vi "Sync_Afterwards.vi"(2 "Analogue Data":dbl[][](array[numeric]) format="%.3f", 4 "LDA Data":dbl[][](array[numeric]) format="%.3f") -> (0 "Eng Values":dbl[][](array[numeric]) format="%.2f")   [LabVIEW 2011]
uses:
  Globals/LDA_meas_global_1.vi
  Globals/Meas_global.vi
  Globals/Dynamic_call_global.ph.vi
panel:
  out "Array":string[](array[string])
  out "Delay (ms)":dbl=13.0 format="%.2f"
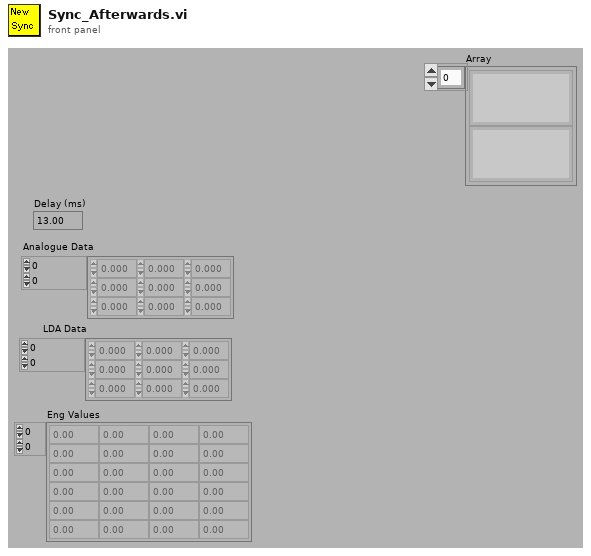
[diagram p1: front panel]
types:
  T1 = typedef "Analysis_info_cluster.ctl" = cluster{"Colour":u32, "Inst type":T2, "Inst name":string, "Symbol":string, "Code name":string, "Extra Info":string, "Inst Array":T3, "Index":i32, "Voltage Index":i32, "Extra Titles":string[], "Extra Values":string[], "Eng Values":dbl[], "Time (ms)":dbl[], "TT / Voltage":dbl[], "U":dbl, "u^2":dbl, "u^3":dbl, "u^4":dbl, "Skew_u":dbl, "Kurt_u":dbl, "Mean % Err":dbl, "% u'/U":dbl}
  T2 = typedef "Inst_type.ctl" = enum16{"Propeller anemometer", "Raw voltage", "Pressure Transducer", "Pitot-static tube", "Preston tube", "Hot wire", "Cross wire 1", "Cross wire 2", "Generic Linear", "Generic Polynomial", "Generic BackPoly", "Fast FID", "Thermocouple", "Cold wire", "Pulsed Wire", "LDA Vel", "LDA Tran time", "LDA Arr time"}
  T3 = typedef "Instrument_Array.ctl" = enum16{"PWA", "LDA", "Analogue"}
  T4 = typedef "Analysis_type_cluster.ctl" = cluster{"Analysis type":T5, "Indicies":i32[], "Name":string, "Inst Array":T3, "Info index":i32}
  T5 = typedef "Analysis_type_Enum.ctl" = enum16{"Slow Response", "Fast Response", "Weighted Fast Response", "Fast FID", "Weighted Fast FID", "Cross Wire", "Weighted Cross Wire", "Weighted LDA"}
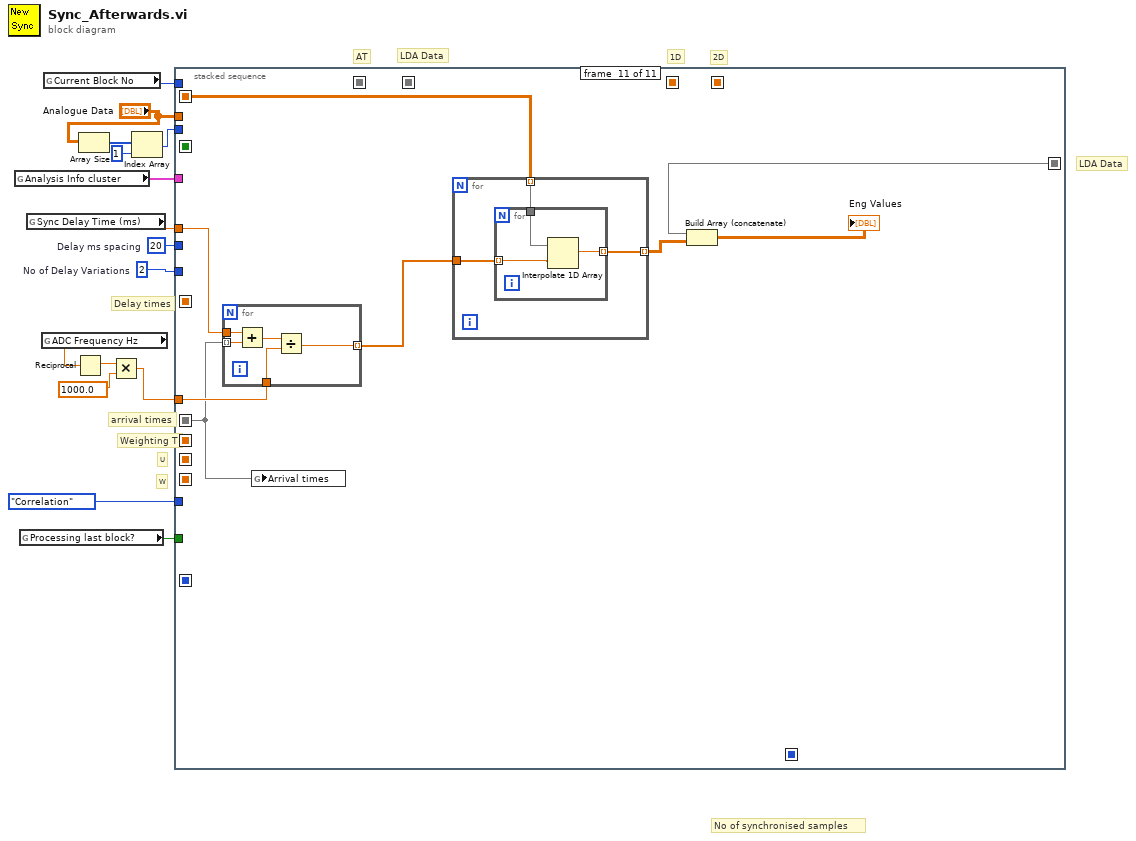
[diagram p0: block diagram]
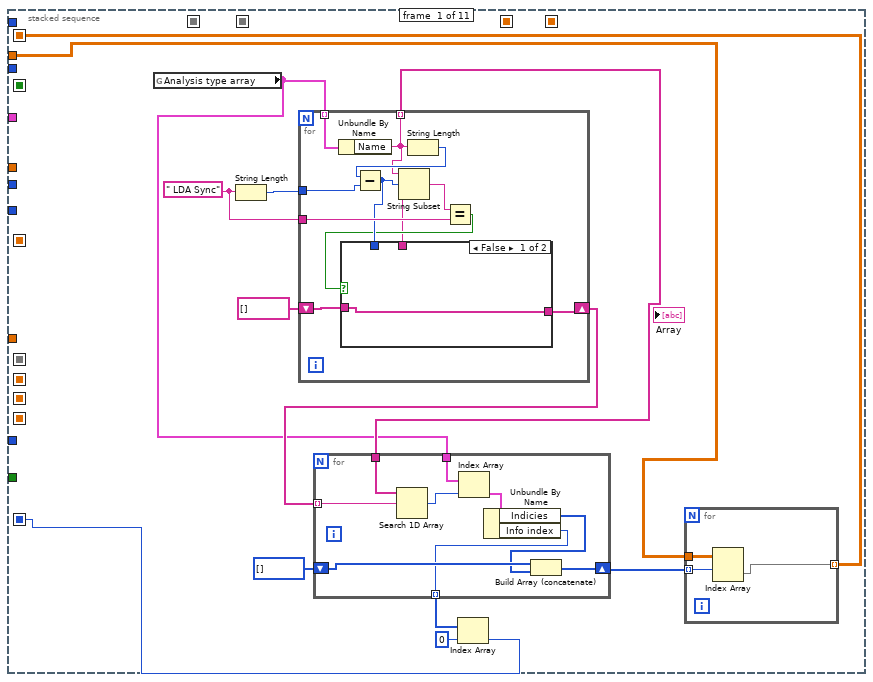
[diagram p2: hidden frame]
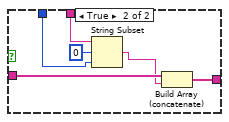
[diagram p3: hidden frame]
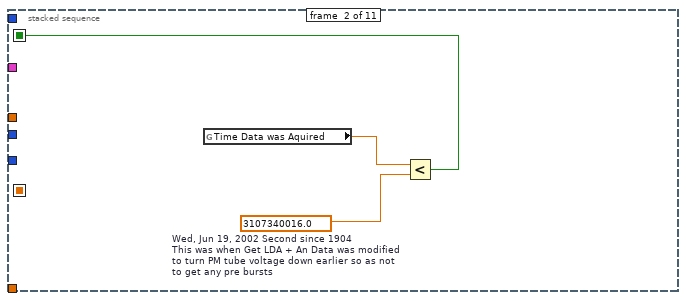
[diagram p4: hidden frame]
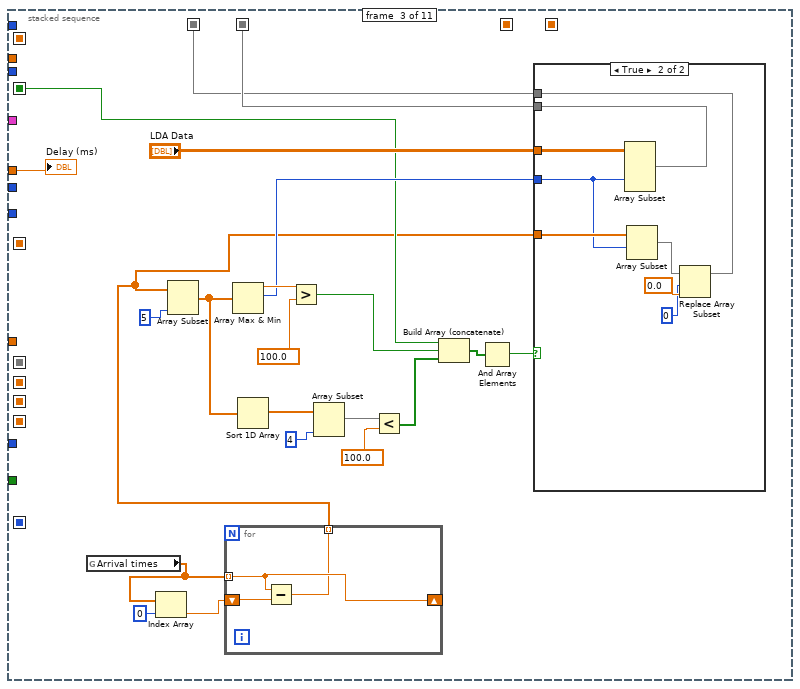
[diagram p5: hidden frame]
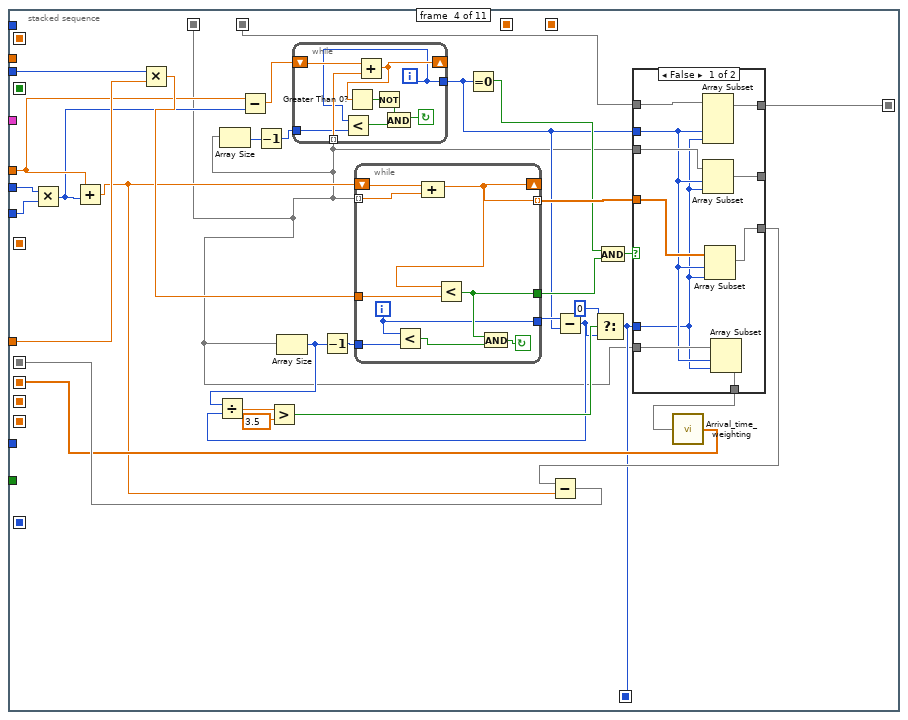
[diagram p7: hidden frame]
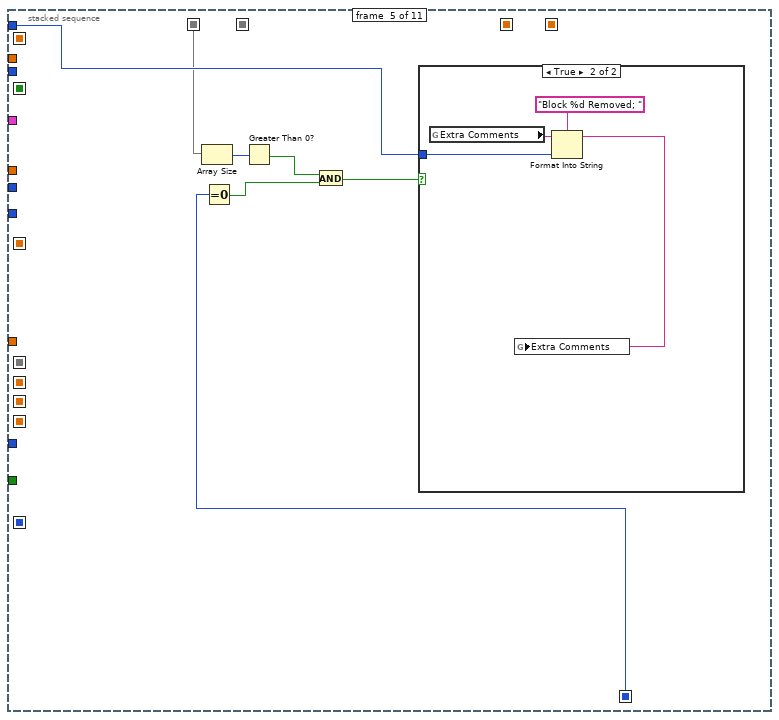
[diagram p9: hidden frame]
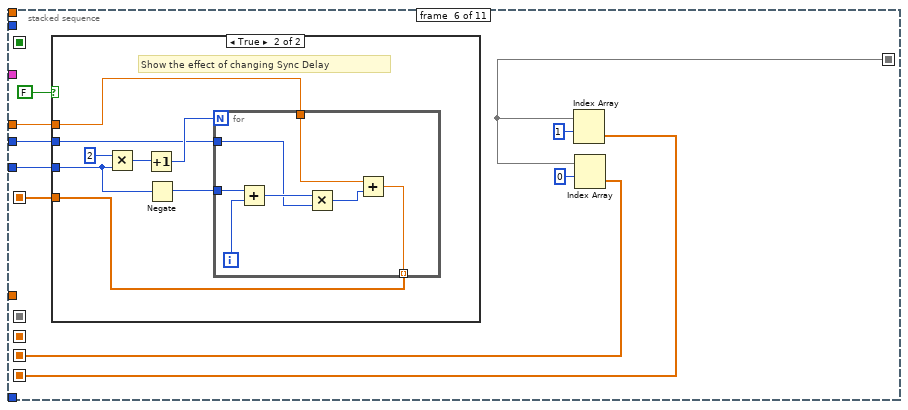
[diagram p11: hidden frame]
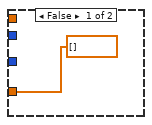
[diagram p12: hidden frame]
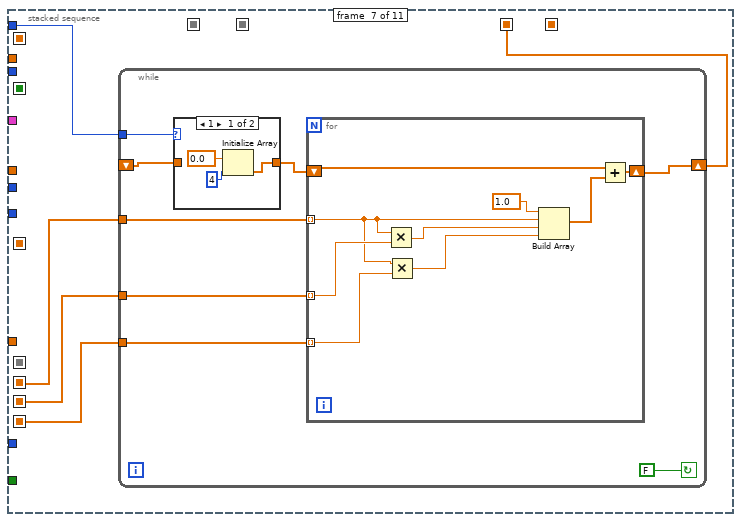
[diagram p13: hidden frame]
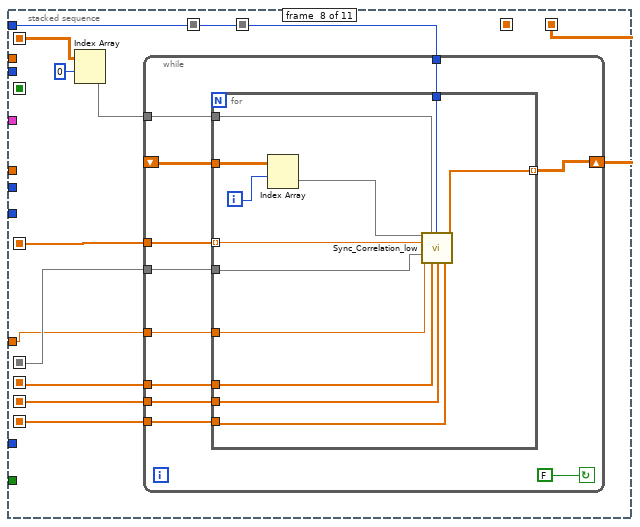
[diagram p15: hidden frame]
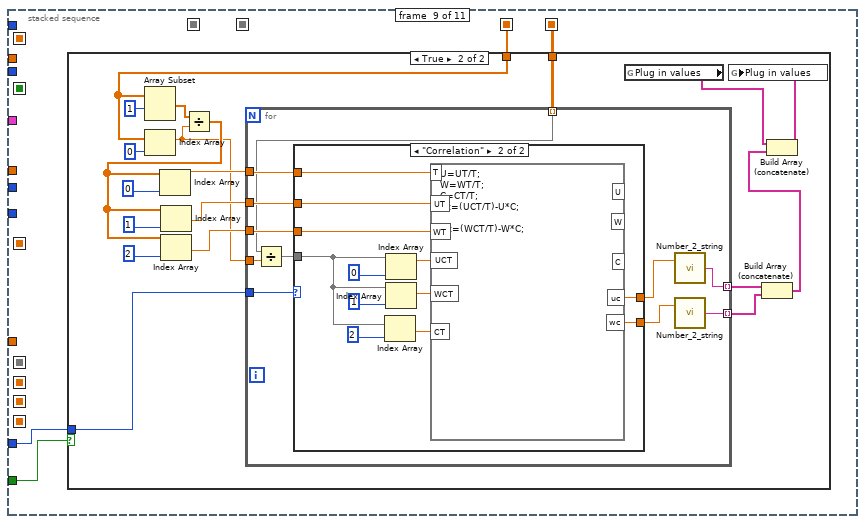
[diagram p16: hidden frame]
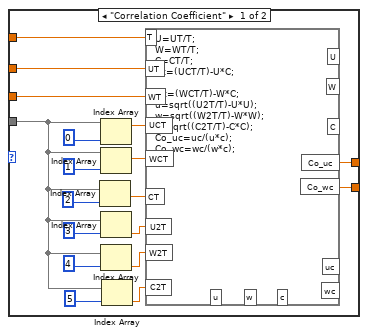
[diagram p18: hidden frame]
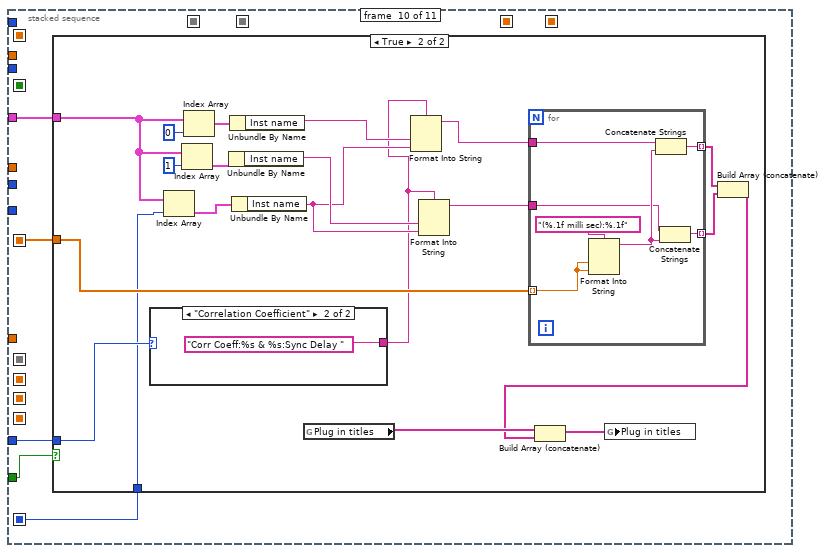
[diagram p19: hidden frame]
diagram:
  w3 = 20  # Delay ms spacing
  w15 = 2  # No of Delay Variations
  # "No of synchronised samples"
  # "AT"
  # "LDA Data"
  # "Delay times"
  # "1D"
  # "2D"
  # "W"
  # "U"
  # "Weighting T"
  # "arrival times"
  # "LDA Data"
  n1 = global read "Meas_global.vi" "Analysis Info cluster"() -> (w1:T1[])
  n2 = global read "Meas_global.vi" "Processing last block?"() -> (w13:bool)
  n3 = global read "LDA_meas_global_1.vi" "Sync Delay Time (ms)"() -> (w8:dbl)
  n4 = global read "LDA_meas_global_1.vi" "ADC Frequency Hz"() -> (w11:dbl)
  n5 = global read "Meas_global.vi" "Current Block No"() -> (w14:i32)
  n6 = Reciprocal(x=w11) -> (1/x=w12:dbl)
  n7 = Array Size(array="Analogue Data") -> (size(s)=w6:i32[])
  n8 = Multiply(x=w12, y=1000.0) -> (x*y=w9:dbl)
  n9 = Index Array(array=w6, index=1 ("Index")) -> (element=w4:i32)
  n10 = stacked-sequence {
    seq-local: [_ _ _ w125 _ _ _ _ _ _ _] -> [_ _ _ _ _ w176 _ _ _ _ w360]
    seq-local: [_ _ _ w122 _ _ _ _ _ _ _] -> [_ _ _ _ _ _ _ w228 _ _ w355]
    seq-local: [_ _ _ w120 _ _ _ _ _ _ _] -> [_ _ _ _ _ _ w201 w229 _ _ _]
    seq-local: [_ _ _ _ _ w175 _ _ _ _ _] -> [_ _ _ _ _ _ w200 w231 _ _ _]
    seq-local: [_ _ _ _ _ w174 _ _ _ _ _] -> [_ _ _ _ _ _ w199 w230 _ _ _]
    seq-local: [_ _ _ _ _ _ _ w226 _ _ _] -> [_ _ _ _ _ _ _ _ w258 _ _]
    seq-local: [_ _ _ _ _ _ w197 _ _ _ _] -> [_ _ _ _ _ _ _ _ w259 _ _]
    seq-local: [_ _ _ _ _ w179 _ _ _ _ _] -> [_ _ _ _ _ _ _ w225 _ w324 _]
    seq-local: [_ _ w69 _ _ _ _ _ _ _ _] -> [_ _ _ w112 _ _ _ _ _ _ _]
    seq-local: [_ _ w68 _ _ _ _ _ _ _ _] -> [_ _ _ w98 w165 _ _ _ _ _ _]
    seq-local: [_ w59 _ _ _ _ _ _ _ _ _] -> [_ _ w65 _ _ _ _ _ _ _ _]
    seq-local: [_ _ _ w102 _ _ _ _ _ _ _] -> [_ _ _ _ w164 _ _ _ _ _ _]
    seq-local: [w17 _ _ _ _ _ _ _ _ _ _] -> [_ _ _ _ _ _ _ _ _ w321 _]
    seq-local: [w16 _ _ _ _ _ _ _ _ _ _] -> [_ _ _ _ _ _ _ w223 _ _ w357]
    tunnel: "Analogue Data" -> [w20 _ _ _ _ _ _ _ _ _ _]
    tunnel: w8 -> [_ _ w66 w114 _ w173 _ _ _ _ w356]
    tunnel: w15 -> [_ _ _ w100 _ w180 _ _ _ _ _]
    tunnel: w14 -> [_ _ _ _ w166 _ w198 w227 _ _ _]
    tunnel: w13 -> [_ _ _ _ _ _ _ _ w260 w325 _]
    tunnel: w9 -> [_ _ _ w119 _ _ _ w224 _ _ w362]
    tunnel: w4 -> [_ _ _ w104 _ _ _ _ _ _ _]
    tunnel: w3 -> [_ _ _ w101 _ w172 _ _ _ _ _]
    tunnel: enum16{"Correlation", "Correlation Coefficient"}."Correlation" -> [_ _ _ _ _ _ _ _ w257 w323 _]
    tunnel: w1 -> [_ _ _ _ _ _ _ _ _ w322 _]
    frame #0 {
      w27 = " LDA Sync" ("Substring")
      n11 = global read "Meas_global.vi" "Analysis type array"() -> (w23:T4[])
      n12 = String Length(string=w27) -> (length=w26:i32)
      n13 = for {
        tunnel: w23 -> [w50] mode=indexing
        tunnel: w26 -> [w48]
        tunnel: w27 -> [w46]
        shift-right: [w42] -> w24
        shift-left: string[] [] -> [w43]
        tunnel: [w41] -> w25 mode=indexing
        n14 = Unbundle By Name(w50) -> ("Name"=w41:string)
        n15 = String Length(string=w41) -> (length=w49:i32)
        n16 = Subtract(x=w49, y=w48) -> (x-y=w45:i32)
        n17 = String Subset(string=w41, offset (0)=w45) -> (substring=w47:string)  [unwired: 1 out]
        n18 = Equal?(x=w47, y=w46) -> (x = y?=w44:bool)
        n19 = case shown="False" w44 {
          tunnel: w41 -> [_ w57]
          tunnel: w45 -> [_ w55]
          tunnel: w43 -> [w51 w54]
          tunnel: [w51 w52] -> w42
          frame False {
          }
          frame True {
            n20 = String Subset(string=w57, offset (0)=0, length (rest)=w55) -> (substring=w53:string)
            n21 = Build Array (concatenate)(w54, w53) -> (w52:string[])
          }
        }
      }
      n22 = for {
        tunnel: w25 -> [w40]
        tunnel: w24 -> [w39] mode=indexing
        tunnel: w23 -> [w38]
        shift-right: [w34] -> w21
        shift-left: i32[] [] -> [w36]
        tunnel: [w32] -> w19 mode=indexing
        n23 = Search 1D Array(1D array=w40, element=w39) -> (index of element=w33:i32)  [unwired: 1 out]
        n24 = Index Array(array=w38, index=w33) -> (element=w37:T4)
        n25 = Unbundle By Name(w37) -> ("Indicies"=w35:i32[], "Info index"=w32:i32)
        n26 = Build Array (concatenate)(w36, w35) -> (w34:i32[])
      }
      n27 = Index Array(array=w19, index=0) -> (element=w17:i32)
      n28 = for {
        tunnel: w21 -> [w31] mode=indexing
        tunnel: w20 -> [w30]
        tunnel: [w29] -> w16 mode=indexing
        n29 = Index Array(array=w30, index (row)=w31) -> (element=w29:dbl[])  [unwired: 1 in]
      }
    }
    frame #1 {
      w60 = 3107340016.0  # Wed, Jun 19, 2002 Second since 1904 This was when Get LDA + An Data was modified to turn PM tube voltage down earlier so as not to get any pre bursts
      n30 = global read "Meas_global.vi" "Time Data was Aquired"() -> (w58:dbl)
      n31 = Less?(x=w58, y=w60) -> (x < y?=w59:bool)
    }
    frame #2 {
      n32 = global read "LDA_meas_global_1.vi" "Arrival times"() -> (w62:dbl[])
      n33 = Index Array(array=w62, index=0) -> (element=w63:dbl)
      n34 = for {
        shift-right: [w84] -> _
        shift-left: w63 -> [w85]
        tunnel: w62 -> [w84] mode=indexing
        tunnel: [w83] -> w61 mode=indexing
        n35 = Subtract(x=w84, y=w85) -> (x-y=w83:dbl)
      }
      n36 = Array Subset(array=w61, length=5 ("Array Length")) -> (w79:dbl[])  [unwired: 1 in]
      n37 = Array Max & Min(array=w79) -> (max value=w81:dbl, max index (indices)=w71:i32)  [unwired: 2 out]
      n38 = Sort 1D Array(array=w79) -> (sorted array=w77:dbl[])
      n39 = Greater?(x=w81, y=100.0) -> (0:w73:bool)
      n40 = Array Subset(array=w77, length=4 ("Array Length")) -> (w76:dbl[])  [unwired: 1 in]
      n41 = Less?(x=w76, y=100.0) -> (x < y?=w74:bool[])
      n42 = Build Array (concatenate)(w65, w73, w74) -> (w72:bool[])
      n43 = And Array Elements(Boolean array=w72) -> (logical AND=w67:bool)
      n44 = case shown="True" w67 {
        tunnel: w71 -> [_ w88]
        tunnel: "LDA Data" -> [w86 w95]
        tunnel: [w86 w94] -> w69
        tunnel: w61 -> [w87 w93]
        tunnel: [w87 w89] -> w68
        frame False {
        }
        frame True {
          n45 = Array Subset(array=w95, index (col)=w88) -> (w94:dbl[][])  [unwired: 3 in]
          n46 = Array Subset(array=w93, index=w88) -> (w92:dbl[])  [unwired: 1 in]
          n47 = Replace Array Subset(array=w92, new element=0.0 ("Element Data"), index=0 ("Index")) -> (w89:dbl[])
        }
      }
      "Delay (ms)" <- w66
    }
    frame #3 {
      n48 = Multiply(x=w101, y=w100) -> (x*y=w99:i32)
      n49 = Add(x=w114, y=w99) -> (x+y=w118:dbl)
      n50 = Multiply(x=w104, y=w119) -> (x*y=w126:dbl)
      n51 = Array Size(array=w98) -> (size(s)=w97:i32)
      n52 = Subtract(x=w114, y=w99) -> (x-y=w113:dbl)
      n53 = Decrement(x=w97) -> (x-1=w96:i32)
      n54 = Array Size(array=w98) -> (size(s)=w107:i32)
      n55 = while {
        tunnel: [w138] -> w110
        tunnel: w98 -> [w140] mode=indexing
        shift-left: w113 -> [w145]
        shift-right: [w144] -> _
        tunnel: w96 -> [w137]
        i -> [w138]
        stop <- w141 continue-if-true
        n56 = Less?(x=w138, y=w137) -> (x < y?=w139:bool)
        n57 = Add(x=w145, y=w140) -> (x+y=w144:dbl)
        n58 = Greater Than 0?(x=w144) -> (x > 0?=w143:bool)
        n59 = Not(x=w143) -> (.not. x?=w142:bool)
        n60 = And(x=w142, y=w139) -> (x .and. y?=w141:bool)
      }
      n61 = Decrement(x=w107) -> (x-1=w127:i32)
      n62 = while {
        tunnel: [w128] -> w124 mode=indexing
        tunnel: [w129] -> w111
        tunnel: [w130] -> w117
        tunnel: w126 -> [w133]
        tunnel: w127 -> [w134]
        tunnel: w98 -> [w135] mode=indexing
        shift-left: w118 -> [w136]
        shift-right: [w128] -> _
        i -> [w129]
        stop <- w131 continue-if-true
        n63 = Less?(x=w129, y=w134) -> (x < y?=w132:bool)
        n64 = Compound Arithmetic op=ADD(w136, w135) -> (w128:dbl)
        n65 = Less?(x=w128, y=w133) -> (x < y?=w130:bool)
        n66 = And(x=w130, y=w132) -> (x .and. y?=w131:bool)
      }
      n67 = Equal To 0?(x=w110) -> (x = 0?=w116:bool)
      n68 = Subtract(x=w111, y=w110) -> (x-y=w103:i32)
      n69 = Divide(x=w107, y=w103) -> (x/y=w108:dbl)
      n70 = Greater?(x=w108, y=3.5) -> (0:w106:bool)
      n71 = Select(t=0, s=w106, f=w103) -> (s? t:f=w102:i32)
      n72 = And(x=w116, y=w117) -> (x .and. y?=w115:bool)
      n73 = case shown="False" w115 {
        tunnel: [w155 w158] -> w123
        tunnel: w102 -> [w147 _]
        tunnel: w112 -> [w154 w159]
        tunnel: [w153 w159] -> w125
        tunnel: w124 -> [w152 w158]
        tunnel: w98 -> [w151 w157]
        tunnel: [w150 w157] -> w121
        tunnel: w110 -> [w148 _]
        tunnel: w98 -> [w149 w156]
        tunnel: [w146 w156] -> _
        frame False {
          n74 = Array Subset(array=w154, index (col)=w148, length (col)=w147) -> (w153:dbl[][])  [unwired: 2 in]
          n75 = Array Subset(array=w149, index=w148, length=w147) -> (w146:dbl[])
          n76 = Array Subset(array=w152, index=w148, length=w147) -> (w155:dbl[])
          n77 = Array Subset(array=w151, index=w148, length=w147) -> (w150:dbl[])
        }
        frame True {
        }
      }
      n78 = Subtract(x=w123, y=w118) -> (x-y=w122:dbl[])
      n79 = call "Arrival_time_weighting.vi"("Arrival times"=w121) -> ("Weighting"=w120:dbl[])
    }
    frame #4 {
      n80 = Array Size(array=w165) -> (size(s)=w163:i32)
      n81 = Equal To 0?(x=w164) -> (x = 0?=w161:bool)
      n82 = Greater Than 0?(x=w163) -> (x > 0?=w162:bool)
      n83 = And(x=w162, y=w161) -> (x .and. y?=w160:bool)
      n84 = case shown="True" w160 {
        tunnel: w166 -> [_ w170]
        frame False {
        }
        frame True {
          n85 = global read "Meas_global.vi" "Extra Comments"() -> (w168:string)
          n86 = Format Into String(format string="Block %d Removed; " ("Format String"), initial string=w168, w170) -> (resulting string=w167:string)  [unwired: 1 in, 1 out]
          n87 = global write "Meas_global.vi" "Extra Comments"(w167) -> ()
        }
      }
    }
    frame #5 {
      n88 = case shown="True" FALSE {
        tunnel: w180 -> [_ w186]
        tunnel: [dbl[] [] w184] -> w179
        tunnel: w173 -> [_ w183]
        tunnel: w172 -> [_ w182]
        frame False {
        }
        frame True {
          # "Show the effect of changing Sync Delay"
          n89 = Multiply(x=2, y=w186) -> (x*y=w188:i32)
          n90 = Increment(x=w188) -> (x+1=w187:i32)
          n91 = Negate(x=w186) -> (-x=w185:i32)
          n92 = for {
            N: w187 -> [_]
            tunnel: w185 -> [w196]
            tunnel: w183 -> [w194]
            tunnel: [w193] -> w184 mode=indexing
            tunnel: w182 -> [w190]
            i -> [w195]
            n93 = Add(x=w196, y=w195) -> (x+y=w192:i32)
            n94 = Multiply(x=w192, y=w190) -> (x*y=w191:i32)
            n95 = Add(x=w194, y=w191) -> (x+y=w193:dbl)
          }
        }
      }
      n96 = Index Array(array=w176, index (row)=1 ("Index")) -> (element=w174:dbl[])  [unwired: 1 in]
      n97 = Index Array(array=w176, index (row)=0 ("Index")) -> (element=w175:dbl[])  [unwired: 1 in]
    }
    frame #6 {
      n98 = while {
        tunnel: w198 -> [w203]
        tunnel: w199 -> [w207]
        tunnel: w200 -> [w208]
        tunnel: w201 -> [w209]
        shift-left: _ -> [w205]
        shift-right: [w204] -> w197
        stop <- FALSE continue-if-true
        n99 = case shown="1" w203 {
          tunnel: [w210 w213] -> w206
          tunnel: w205 -> [_ w213]
          frame 1 {
            n100 = Initialize Array(0.0 ("Element Data"), 4 ("Dimension Size")) -> (w210:dbl[])
          }
          frame 2, Default {
          }
        }
        n101 = for {
          shift-right: [w221] -> w204
          shift-left: w206 -> [w222]
          tunnel: w209 -> [w217] mode=indexing
          tunnel: w208 -> [w220] mode=indexing
          tunnel: w207 -> [w216] mode=indexing
          n102 = Multiply(x=w217, y=w220) -> (x*y=w219:dbl)
          n103 = Multiply(x=w217, y=w216) -> (x*y=w215:dbl)
          n104 = Build Array(1.0 ("Input Element"), w217, w219, w215) -> (w214:dbl[])
          n105 = Add(x=w222, y=w214) -> (x+y=w221:dbl[])
        }
      }
    }
    frame #7 {
      n106 = Index Array(array=w223, index (row)=0 ("Index")) -> (element=w232:dbl[])  [unwired: 1 in]
      n107 = while {
        tunnel: w225 -> [w235]
        shift-left: _ -> [w237]
        shift-right: [w236] -> w226
        tunnel: w227 -> [w238]
        tunnel: w228 -> [w239]
        tunnel: w229 -> [w240]
        tunnel: w230 -> [w241]
        tunnel: w231 -> [w242]
        tunnel: w232 -> [w243]
        tunnel: w224 -> [w244]
        stop <- FALSE continue-if-true
        n108 = for {
          tunnel: w239 -> [w256]
          tunnel: w244 -> [w255]
          tunnel: w243 -> [w254]
          tunnel: w242 -> [w253]
          tunnel: w241 -> [w252]
          tunnel: w240 -> [w251]
          tunnel: [w250] -> w236 mode=indexing
          tunnel: w238 -> [w249]
          tunnel: w237 -> [w247]
          tunnel: w235 -> [w245] mode=indexing
          i -> [w246]
          n109 = Index Array(array=w247, index (row)=w246) -> (element=w248:dbl[])  [unwired: 1 in]
          n110 = call "Sync_Correlation_low.vi"("Shift In"=w248, "Analogue Data"=w254, "Block No"=w249, "Delay (ms)"=w245, "Arrival Times"=w256, "Delta T (ms)"=w255, "T"=w251, "U"=w253, "W"=w252) -> ("Shift Out"=w250:dbl[])  [unwired: 6 out]
        }
      }
    }
    frame #8 {
      n111 = case shown="True" w260 {
        tunnel: w259 -> [_ w277]
        tunnel: w258 -> [_ w267]
        tunnel: w257 -> [_ w265]
        frame False {
        }
        frame True {
          n112 = Array Subset(array=w277, index=1 ("Array Index")) -> (w276:dbl[])  [unwired: 1 in]
          n113 = Index Array(array=w277, index=0 ("Index")) -> (element=w268:dbl)
          n114 = Divide(x=w276, y=w268) -> (x/y=w272:dbl[])
          n115 = Index Array(array=w272, index=0) -> (element=w271:dbl)
          n116 = Index Array(array=w272, index=1) -> (element=w270:dbl)
          n117 = Index Array(array=w272, index=2) -> (element=w269:dbl)
          n118 = for {
            tunnel: w271 -> [w288]
            tunnel: w270 -> [w290]
            tunnel: w269 -> [w289]
            tunnel: w268 -> [w287]
            tunnel: w267 -> [w286] mode=indexing
            tunnel: w265 -> [w284]
            tunnel: [w281] -> w263 mode=indexing
            tunnel: [w280] -> w262 mode=indexing
            n119 = Divide(x=w286, y=w287) -> (x/y=w285:dbl[])
            n120 = case shown="\"Correlation\"" w284 {
              tunnel: w290 -> [w305 w317]
              tunnel: w289 -> [w304 w316]
              tunnel: w288 -> [w300 w312]
              tunnel: w285 -> [w296 w311]
              tunnel: [w292 w310] -> w283
              tunnel: [w291 w309] -> w282
              frame "Correlation Coefficient" {
                n121 = Index Array(array=w296, index=2) -> (element=w301:dbl)
                n122 = Index Array(array=w296, index=0) -> (element=w303:dbl)
                n123 = Index Array(array=w296, index=1) -> (element=w302:dbl)
                n124 = Index Array(array=w296, index=3) -> (element=w293:dbl)
                n125 = Index Array(array=w296, index=4) -> (element=w294:dbl)
                n126 = Index Array(array=w296, index=5) -> (element=w295:dbl)
                n127 = formula code="U=UT/T;\nW=WT/T;\nC=CT/T;\nuc=(UCT/T)-U*C;\n\nwc=(WCT/T)-W*C;\nu=sqrt((U2T/T)-U*U);\nw=sqrt((W2T/T)-W*W);\nc=sqrt((C2T/T)-C*C);\nCo_uc=uc/(u*c);\nCo_wc=wc/(w*c);"("T"=w300, "UT"=w305, "WT"=w304, "WCT"=w302, "CT"=w301, "UCT"=w303, "U2T"=w293, "W2T"=w294, "C2T"=w295) -> ("Co_uc"=w292:dbl, "Co_wc"=w291:dbl)  [unwired: 8 out]
              }
              frame "Correlation" {
                n128 = Index Array(array=w311, index=2) -> (element=w313:dbl)
                n129 = Index Array(array=w311, index=0) -> (element=w315:dbl)
                n130 = Index Array(array=w311, index=1) -> (element=w314:dbl)
                n131 = formula code="U=UT/T;\nW=WT/T;\nC=CT/T;\nuc=(UCT/T)-U*C;\n\nwc=(WCT/T)-W*C;"("T"=w312, "UT"=w317, "WT"=w316, "WCT"=w314, "CT"=w313, "UCT"=w315) -> ("uc"=w310:dbl, "wc"=w309:dbl)  [unwired: 3 out]
              }
            }
            n132 = call "Number_2_string.vi"("number"=w283) -> ("String"=w280:string)  [unwired: 1 in]
            n133 = call "Number_2_string.vi"("number"=w282) -> ("String"=w281:string)  [unwired: 1 in]
          }
          n134 = global read "Dynamic_call_global.ph.vi" "Plug in values"() -> (w264:string[])
          n135 = Build Array (concatenate)(w262, w263) -> (w261:string[])
          n136 = Build Array (concatenate)(w264, w261) -> (w266:string[])
          n137 = global write "Dynamic_call_global.ph.vi" "Plug in values"(w266) -> ()
        }
      }
    }
    frame #9 {
      n138 = case shown="True" w325 {
        tunnel: w324 -> [_ w338]
        tunnel: w323 -> [_ w329]
        tunnel: w322 -> [_ w327]
        tunnel: w321 -> [_ w326]
        frame False {
        }
        frame True {
          n139 = case shown="\"Correlation Coefficient\"" w329 {
            tunnel: ["Correlation:%s & %s:Sync Delay " ("Format String") "Corr Coeff:%s & %s:Sync Delay " ("Format String")] -> w328
            frame "Correlation" {
            }
            frame "Correlation Coefficient" {
            }
          }
          n140 = Index Array(array=w327, index=w326) -> (element=w343:T1)
          n141 = Index Array(array=w327, index=1 ("Index")) -> (element=w339:T1)
          n142 = Index Array(array=w327, index=0 ("Index")) -> (element=w340:T1)
          n143 = Unbundle By Name(w339) -> ("Inst name"=w336:string)
          n144 = Unbundle By Name(w340) -> ("Inst name"=w337:string)
          n145 = Unbundle By Name(w343) -> ("Inst name"=w335:string)
          n146 = global read "Dynamic_call_global.ph.vi" "Plug in titles"() -> (w345:string[])
          n147 = Format Into String(format string=w328, w337, w335) -> (resulting string=w334:string)  [unwired: 2 in, 1 out]
          n148 = Format Into String(format string=w328, w336, w335) -> (resulting string=w333:string)  [unwired: 2 in, 1 out]
          n149 = for {
            tunnel: w338 -> [w353] mode=indexing
            tunnel: w334 -> [w351]
            tunnel: w333 -> [w350]
            tunnel: [w349] -> w332 mode=indexing
            tunnel: [w348] -> w331 mode=indexing
            n150 = Format Into String(format string="(%.1f milli sec):%.1f" ("Format String"), w353, w353) -> (resulting string=w352:string)  [unwired: 2 in, 1 out]
            n151 = Concatenate Strings(w351, w352) -> (w349:string)
            n152 = Concatenate Strings(w350, w352) -> (w348:string)
          }
          n153 = Build Array (concatenate)(w332, w331) -> (w330:string[])
          n154 = Build Array (concatenate)(w345, w330) -> (w344:string[])
          n155 = global write "Dynamic_call_global.ph.vi" "Plug in titles"(w344) -> ()
        }
      }
    }
    frame #10 {
      n156 = for {
        tunnel: w356 -> [w367]
        tunnel: w355 -> [w366] mode=indexing
        tunnel: w362 -> [w365]
        tunnel: [w364] -> w361 mode=indexing
        n157 = Add(x=w367, y=w366) -> (x+y=w363:dbl)
        n158 = Divide(x=w363, y=w365) -> (x/y=w364:dbl)
      }
      n159 = global write "LDA_meas_global_1.vi" "Arrival times"(w355) -> ()
      n160 = for {
        tunnel: w357 -> [w370] mode=indexing
        tunnel: w361 -> [w369]
        tunnel: [w368] -> w359 mode=indexing
        n161 = for {
          tunnel: w370 -> [w373]
          tunnel: w369 -> [w372] mode=indexing
          tunnel: [w371] -> w368 mode=indexing
          n162 = Interpolate 1D Array(1:w372, 2:w373) -> (0:w371:dbl)
        }
      }
      n163 = Build Array (concatenate)(w360, w359) -> (→"Eng Values":dbl[][])
    }
  }
